vi "Check Mouse Up.vi"(8 "error in":errorcluster) -> (0 "error out":errorcluster, 3 "Up?":bool)   [LabVIEW 2015]
uses:
  <vilib>/Utility/inputDevices.llb/mouseAcquire.vi
  <vilib>/Utility/inputDevices.llb/closeMouse.vi
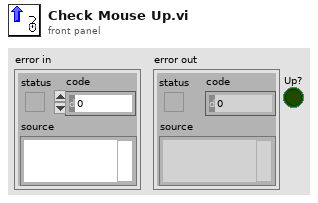
[diagram p1: front panel]
types:
  T1 = cluster{"button 1":bool, "button 2":bool, "button 3":bool, "button 4":bool}
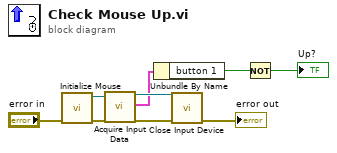
[diagram p0: block diagram]
diagram:
  n1 = call <vilib>:"Initialize Mouse.vi"("error in (no error)"="error in") -> ("error out"=w4:errorcluster, "device ID"=w5:refnum<k1>)  [unwired: 9 in]
  n2 = call-poly <vilib>:"Acquire Input Data.vi"("device ID"=w5, "error in (no error)"=w4) -> ("device ID"=w9:refnum<k1>, "button info"=w6:T1, "error out"=w8:errorcluster)  [unwired: 14 in, 1 out]
  n3 = Unbundle By Name(w6) -> ("button 1"=w7:bool)
  n4 = call-poly <vilib>:"Close Input Device.vi"("error in (no error)"=w8, "device ID"=w9) -> ("error out"=→"error out":errorcluster)  [unwired: 8 in]
  n5 = Not(x=w7) -> (.not. x?=→"Up?":bool)
